vi "Instrument Type ID.vi"() -> (1 "instrument type id":string="niDCPower")   [LabVIEW 2020, in "MeasurementLink niDCPower.lvlib" / "Instrument.lvclass"]
uses:
  Instrument/Instrument.lvclass
  Instrument/Instrument.lvclass/Instrument.ctl
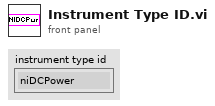
[diagram p1: front panel]
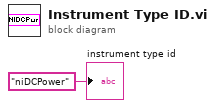
[diagram p0: block diagram]
diagram:
  "instrument type id" <- "niDCPower"
